vi "rs3 Advanced set Color control3.vi"(8 "error in (no error)":errorcluster, 10 "ST Color Control":T1, 11 "device in":u64) -> (0 "error out":errorcluster, 1 "error":u64, 3 "Dev out":u64)   [LabVIEW 2017, in "libRealSense3.lvlib"]
doc: "This sets some register that affect the depth calculations"
uses:
  <vilib>/addons/RealSense/libRealSense3.lvlib
  Users/Greg McKaskle/Downloads/librealsense-1.12.1/librealsense-1.12.1/bin/Win32/realsense-d.dll
panel:
  # "RS3 Adv. Get Color Control 2"
  # "(C) 2017 Intel Corp.,  AGJ"
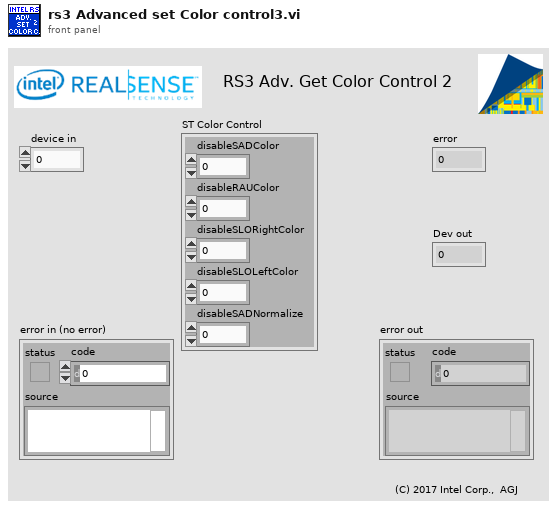
[diagram p1: front panel]
types:
  T1 = cluster{"disableSADColor":u32, "disableRAUColor":u32, "disableSLORightColor":u32, "disableSLOLeftColor":u32, "disableSADNormalize":u32}
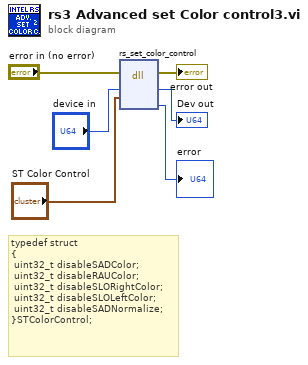
[diagram p0: block diagram]
diagram:
  # "typedef struct\n{\n\tuint32_t disableSADColor;\n\tuint32_t disableRAUColor;\n\tuint32_t disableSLORightColor;\n\tuint32_t disableSLOLeftColor;\n\tuint32_t disableSADNormalize;\n}STColorControl;"
  n1 = dll-call lib="C:/Users/Greg McKaskle/Downloads/librealsense-1.12.1/librealsense-1.12.1/bin/Win32/realsense-d.dll" fn="rs_set_color_control"(error in="error in (no error)", "device"="device in", "ST Color Control"="ST Color Control") -> (error out=→"error out":errorcluster, "device"=→"Dev out":u64, "error"=→"error":u64)  [unwired: 5 in, 1 out]
